vi "All Laser Emission Off.vi"   [LabVIEW 2016]
uses:
  Hardware Configuration/Hardware Configuration Controls/Device Type.ctl
  Device Manager/Common Device Queue/Common Device Controls/Common Device Actions.ctl
types:
  T1 = typedef "Device Type.ctl" = enum16{"AOTF", "Camera", "Deformable Mirror", "Laser", "Shutter", "Stage", "Waveform", "FPGA", "Email", "Filter Wheel"}
  T2 = typedef "Common Device Actions.ctl" = enum16{"Specific Action", "Open Front Panel", "Close Front Panel", "Quit", "Quit All"}
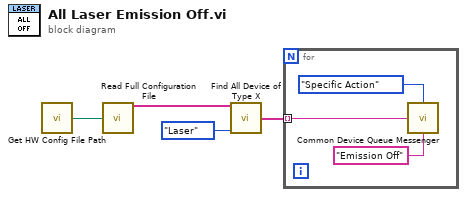
[diagram p0: block diagram]
diagram:
  n1 = call "Get HW Config File Path.vi"() -> ("File Path"=w1:path)  [unwired: 14 in, 1 out]
  n2 = call "Read Full Configuration File.vi"("Config File Path"=w1) -> ("Unique Notifier Names"=w4:string[])  [unwired: 11 in, 3 out]
  n3 = call "Find All Device of Type X.vi"("Unique Notifier Names"=w4, "Device Type"=Device_Type."Laser") -> ("Running Devices"=w2:string[])  [unwired: 12 in, 1 out]
  n4 = for {
    tunnel: w2 -> [w7] mode=indexing
    n5 = call "Common Device Queue Messenger.vi"("Common Action"=Common_Device_Actions."Specific Action", "Notifier Name"=w7, "Specific Action"="Emission Off") -> ()  [unwired: 12 in, 1 out]
  }
